vi "Update Remote Node Info.vi"(8 "error in (no error)":errorcluster, 10 "Discovery":T1, 11 "DiscoveryService in":refnum<class "DiscoveryService.lvclass">) -> (0 "error out":errorcluster, 3 "DiscoveryService out":refnum<class "DiscoveryService.lvclass">)   [LabVIEW 2020, in "Vecto.lvlib" / "DiscoveryService.lvclass"]
uses:
  DiscoveryService.lvclass
  proto/Discovery/Data.ctl
  proto/Service/Data.ctl
  proto/ServiceType/Enumeration.ctl
  DiscoveryService.lvclass/DiscoveryService.ctl
  <vilib>/Utility/miscctls.llb/LVMapReplaceAction.ctl
  proto/ServiceType/ServiceType.lvlib
  proto/Service/Service.lvlib
  proto/Discovery/Discovery.lvlib
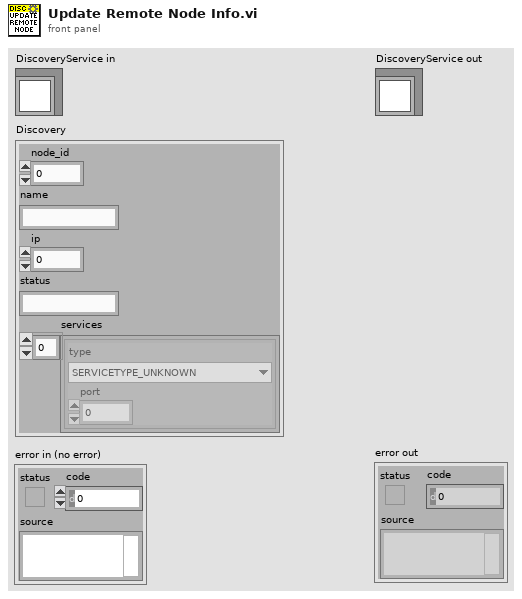
[diagram p1: front panel]
types:
  T1 = typedef "Discovery.lvlib/Data.ctl" = cluster{"node_id":u32, "name":string, "ip":u32, "status":string, "services":T2[]}
  T2 = typedef "Service.lvlib/Data.ctl" = cluster{"type":T3, "port":i32}
  T3 = typedef "ServiceType.lvlib/Enumeration.ctl" = enum16{"SERVICETYPE_UNKNOWN", "SERVICETYPE_TCPSERVER", "SERVICETYPE_HTTPSERVER"}
  T4 = typedef "LVMapReplaceAction.ctl" = enum32{"Modify Entry only if found", "Add or Modify Entry", "Delete Entry"}
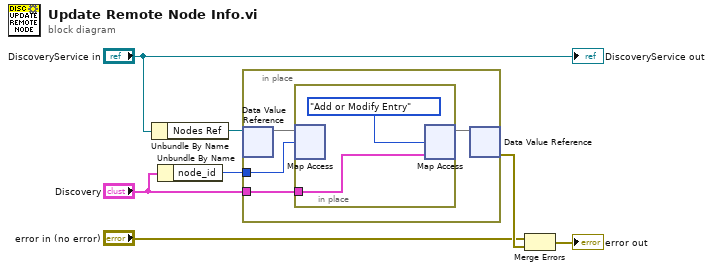
[diagram p0: block diagram]
diagram:
  n1 = Unbundle By Name("DiscoveryService in") -> ("Nodes Ref"=w7:refnum<data-value>)
  n2 = Unbundle By Name("Discovery") -> ("node_id"=w6:u32)
  n3 = in-place {
    in-place-border: w6 -> [w10]
    in-place-border: "Discovery" -> [w9]
    n4 = in-place-dvr #1(w7) -> (w11:map{u32, T1})  [unwired: 1 out]
    n5 = in-place {
      in-place-border: w9 -> [w12]
      n6 = in-place-map #2(w11, w10) -> ()  [unwired: 1 in, 2 out]
      n7 = in-place-map #2(w12, LVMapReplaceAction."Add or Modify Entry" ("action")) -> (w8:map{u32, T1})  [unwired: 2 out]
    }
    n8 = in-place-dvr #1(w8) -> (w3:errorcluster)  [unwired: 1 out]
  }
  n9 = Merge Errors("error in (no error)", w3) -> (→"error out":errorcluster)
  "DiscoveryService out" <- "DiscoveryService in"
